vi "Get Nodes Recursively.vi"(8 "error in (no error)":errorcluster, 10 "Node Name":string, 11 "Nodes Array in":refnum<k20>[](array[refnum])) -> (0 "error out":errorcluster, 2 "Nodes Array out":refnum<k20>[](array[refnum]))   [LabVIEW 2020, in "LVLIBP CD XML Updater.lvlib" / "Project XML Editor.lvclass"]
uses:
  Project XML Editor.lvclass
  <vilib>/xml/Close Reference(Node).vi
  <resource>/objmgr/DOMUserDefRef.rc
  <vilib>/xml/NI_XML.lvlib
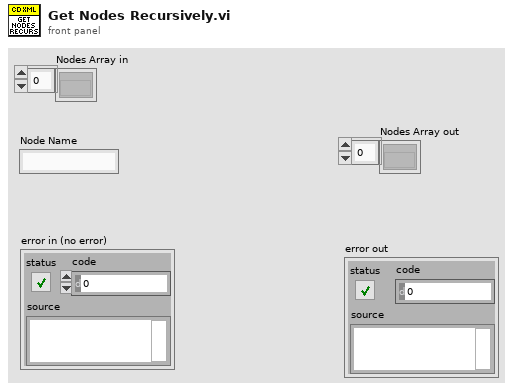
[diagram p1: front panel]
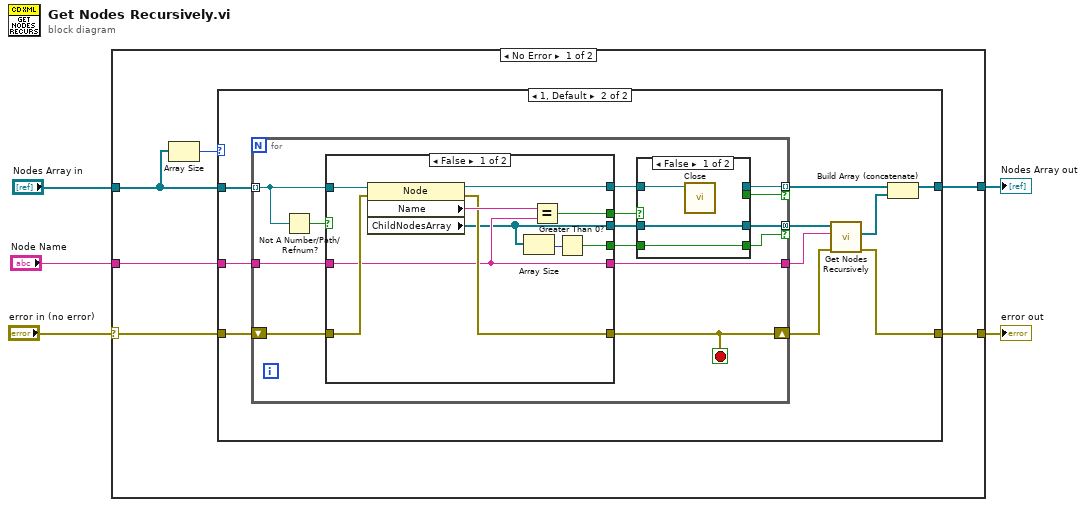
[diagram p0: block diagram]
diagram:
  n1 = case shown="No Error" "error in (no error)" {
    selector: "error in (no error)" -> [w10 _]
    tunnel: "Node Name" -> [w11 _]
    tunnel: "Nodes Array in" -> [w7 _]
    tunnel: [w8 _] -> w3
    tunnel: [w9 _] -> w1
    frame No Error {
      n2 = Array Size(array=w7) -> (size(s)=w6:i32)
      n3 = case shown="1, Default" w6 {
        tunnel: w11 -> [_ w22]
        tunnel: w10 -> [w12 w21]
        tunnel: [w12 w17] -> w9
        tunnel: [_ w13] -> w8
        tunnel: w7 -> [_ w15]
        frame 0 {
        }
        frame 1, Default {
          n4 = for {
            tunnel: w15 -> [w34] mode=indexing
            tunnel: w22 -> [w35]
            tunnel: [w27] -> w20 mode=concatenating if=w25
            shift-right: [w23] -> w18
            shift-left: w21 -> [w36]
            tunnel: [w32] -> w19
            tunnel: [w29] -> w14 mode=indexing if=w24
            stop <- w23 stop-if-true
            n5 = Not A Number/Path/Refnum?(number/path/refnum=w34) -> (NaN/Path/Refnum?=w33:bool)
            n6 = case shown="False" w33 {
              tunnel: w36 -> [w52 w55]
              tunnel: [w46 _] -> w28
              tunnel: w35 -> [w47 w54]
              tunnel: [w51 w56] -> w31
              tunnel: [w50 _] -> w30
              tunnel: [w49 w55] -> w23
              tunnel: w34 -> [w48 w56]
              tunnel: [w47 w54] -> w32
              tunnel: [w44 _] -> w26
              frame False {
                n7 = property class="Node"(reference=w48, error in=w52) -> (reference out=w51:refnum<k20>, error out=w49:errorcluster, "Name"=w53:string, "ChildNodesArray"=w46:refnum<k20>[])
                n8 = Array Size(array=w46) -> (size(s)=w45:i32)
                n9 = Equal?(x=w53, y=w47) -> (x = y?=w50:bool)
                n10 = Greater Than 0?(x=w45) -> (x > 0?=w44:bool)
              }
              frame True {
              }
            }
            n11 = case shown="False" w30 {
              selector: w30 -> [_ w40]
              tunnel: w31 -> [w39 w43]
              tunnel: [_ w43] -> w29
              tunnel: w28 -> [w38 w42]
              tunnel: [w38 w42] -> w27
              tunnel: w26 -> [w37 w41]
              tunnel: [w37 w41] -> w25
              tunnel: [_ w40] -> w24
              frame False {
                n12 = call-poly <vilib>:"Close.vi"("node"=w39) -> ()  [unwired: 8 in, 1 out]
              }
              frame True {
              }
            }
          }
          n13 = call "Get Nodes Recursively.vi"("error in (no error)"=w18, "Node Name"=w19, "Nodes Array in"=w20) -> ("error out"=w17:errorcluster, "Nodes Array out"=w16:refnum<k20>[])  [unwired: 7 in]
          n14 = Build Array (concatenate)(w14, w16) -> (w13:refnum<k20>[])
        }
      }
    }
    frame Error {
    }
  }
  "Nodes Array out" <- w3
  "error out" <- w1
